vi "create_instance_by_label.vi"(7 "call constructor?":bool, 8 "error in (no error)":errorcluster, 9 "label":string, 10 "configuration list":T1[](array[typedef])) -> (0 "error out":errorcluster, 3 "GenericPlugin out":refnum<class "GenericComponent.lvclass">)   [LabVIEW 2010, in "GenericComponent.lvclass"]
uses:
  GenericComponent.lvclass
  clusters/plugin_specification.ctl
  ErrorController/ErrorController/class_data.vi
  ErrorController/ErrorController/ErrorController.lvclass
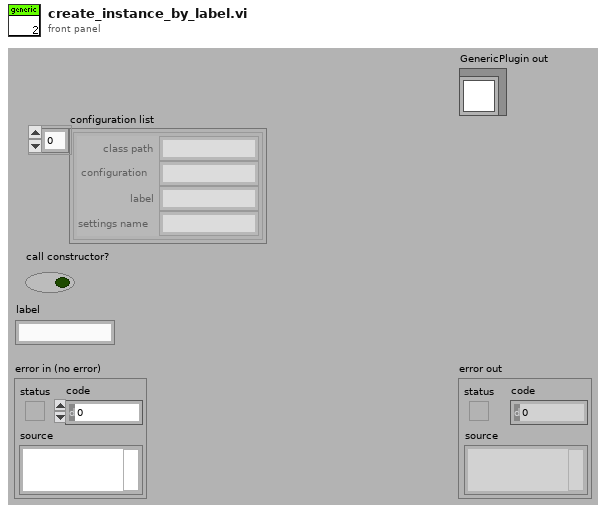
[diagram p1: front panel]
types:
  T1 = typedef "plugin_specification.ctl" = cluster{"class path":string, "configuration":string, "label":string, "settings name":string}
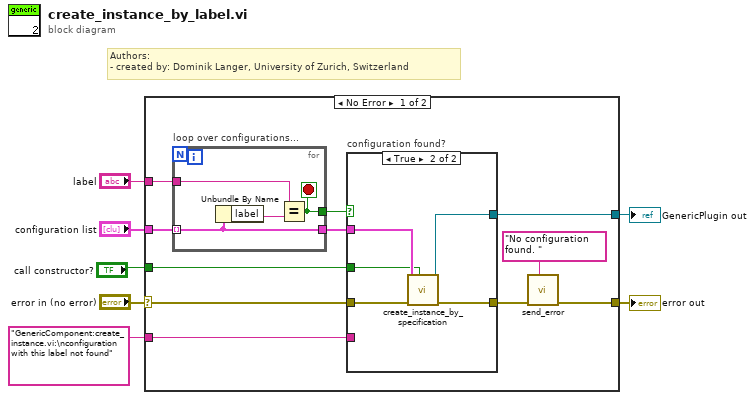
[diagram p0: block diagram]
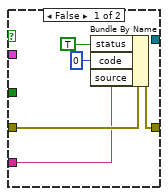
[diagram p2: hidden frame]
diagram:
  # "Authors: \n- created by: Dominik Langer, University of Zurich, Switzerland"
  n1 = case shown="No Error" "error in (no error)" {
    selector: "error in (no error)" -> [w18 w33]
    tunnel: [w10 w33] -> w6
    tunnel: "configuration list" -> [w17 _]
    tunnel: "label" -> [w16 _]
    tunnel: [w15 _] -> w3
    tunnel: "GenericComponent:create_instance.vi:\nconfiguration with this label not found" ("additional message") -> [w13 _]
    tunnel: "call constructor?" -> [w11 _]
    frame No Error {
      n2 = for "loop over configurations..." {
        tunnel: w17 -> [w29] mode=indexing
        tunnel: w16 -> [w32]
        tunnel: [w30] -> w14
        tunnel: [w29] -> w12
        stop <- w30 stop-if-true
        n3 = Unbundle By Name(w29) -> ("label"=w31:string)
        n4 = Equal?(x=w32, y=w31) -> (x = y?=w30:bool)
      }
      n5 = case "configuration found?" shown="True" w14 {
        tunnel: w18 -> [w23 w28]
        tunnel: [w22 w27] -> w9
        tunnel: [_ w25] -> w15
        tunnel: w13 -> [w20 _]
        tunnel: w12 -> [_ w26]
        tunnel: w11 -> [_ w24]
        frame False {
          n6 = Bundle By Name(cluster=w23, "status"=TRUE, "code"=0, "source"=w20) -> (w22:errorcluster)
        }
        frame True {
          n7 = call "create_instance_by_specification.vi"("call constructor?"=w24, "error in (no error)"=w28, "component specification"=w26) -> ("error out"=w27:errorcluster, "GenericPlugin out"=w25:refnum<class "GenericComponent.lvclass">)  [unwired: 6 in, 1 out]
        }
      }
      n8 = call "send_error.vi"("additional message"="No configuration found. ", "error in (no error)"=w9) -> ("error out"=w10:errorcluster)  [unwired: 9 in]
    }
    frame Error {
    }
  }
  "error out" <- w6
  "GenericPlugin out" <- w3
